vi "2025_day5_Task01.vi"() -> ()   [LabVIEW 2025]
uses:
  <userlib>/_OpenG.lib/string/string.llb/openg_string.lvlib
panel:
  out "Task 1":i16
  in  "Switch":bool caption="Ex. Data  vs.  User Data"
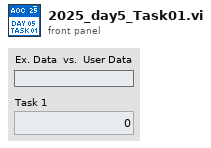
[diagram p1: front panel]
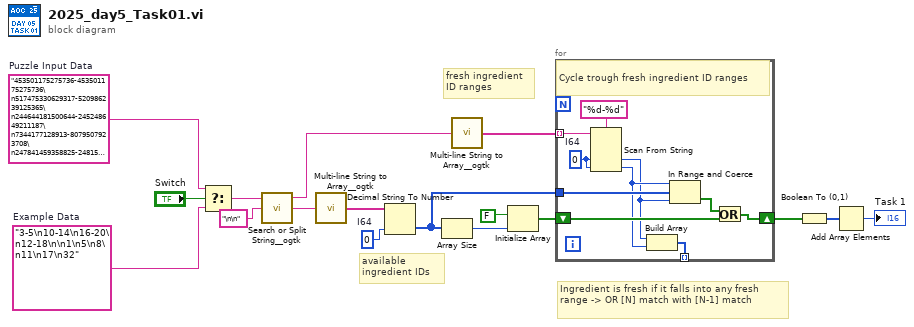
[diagram p0: block diagram]
diagram:
  w1 = "3-5\n10-14\n16-20\n12-18\n\n1\n5\n8\n11\n17\n32"  # Example Data
  w4 = i64 0  # I64
  w16 = "453501175275736-453501175275736\n517475330629317-520986239125365\n244644181500644-245248649211187\n7344177128913-8079507923708\n247841459358825-248157560660015\n417059081741636-417263454551096\n450450656167055-451891555629956\n169036786348951-170691869849947\n102515577547777-103855098233379\n173710182647207-175624825088317\n265859412740011-266721071618589\n526589711508465-531726256938668\n31657887846264-39778138412720\n302893337677460-304531011499720\n91534526078933-98924535693691\n307952023725936-309174375122108\n463113777591287-470890050909438\n101720477800976-103173637373455\n232179792142498-235719322828799\n..."  # Puzzle Input Data
  # "Ingredient is fresh if it falls into any fresh range -> OR [N] match with [N-1] match"
  # "fresh ingredient ID ranges"
  # "available ingredient IDs"
  n1 = Select(t=w16, s="Switch", f=w1) -> (s? t:f=w15:string)
  n2 = call <userlib>:"Search or Split String__ogtk.vi"("search string/char (-)"="\n\n", "string"=w15) -> ("substring after match"=w12:string, "substring before match"=w13:string)  [unwired: 1 in, 1 out]
  n3 = call <userlib>:"Multi-line String to Array__ogtk.vi"("string"=w12) -> ("lines"=w11:string[])
  n4 = Decimal String To Number(string=w11, default (0L)=w4) -> (number=w8:i64[])  [unwired: 1 in, 1 out]
  n5 = Array Size(array=w8) -> (size(s)=w3:i32)
  n6 = call <userlib>:"Multi-line String to Array__ogtk.vi"("string"=w13) -> ("lines"=w2:string[])
  n7 = Initialize Array(FALSE ("line"), w3) -> (w9:bool[])
  n8 = for {
    tunnel: w2 -> [w27] mode=indexing
    tunnel: w8 -> [w25]
    shift-right: [w23] -> w7
    shift-left: w9 -> [w22]
    tunnel: [w18] -> _ mode=indexing
    w21 = i64 0  # I64
    # "Cycle trough fresh ingredient ID ranges"
    n9 = Scan From String(format string="%d-%d", input string=w27, default 1=w21, default 2=w21) -> (output 1=w19:i64, output 2=w20:i64)  [unwired: 2 in, 3 out]
    n10 = Build Array(w19, w20) -> (w18:i64[])
    n11 = In Range and Coerce(upper limit=w20, x=w25, lower limit=w19) -> (In Range?=w24:bool[])  [unwired: 1 out]
    n12 = Or(x=w24, y=w22) -> (x .or. y?=w23:bool[])
  }
  n13 = Boolean To (0,1)(Boolean=w7) -> (0, 1=w6:i16[])
  n14 = Add Array Elements(numeric array=w6) -> (sum=→"Task 1":i16)
